vi "Fetch Measurement (Multiple Point).vi"(0 "VISA resource name":refnum<visa-resource-name>, 5 "Timeout (10000 ms)":u32=10000, 11 "error in (no error)":errorcluster) -> (3 "Go":bool, 4 "VISA resource name out":refnum<visa-resource-name>, 6 "Measurements":dbl[](array[numeric]) format="%#_7g", 10 "Questionable Data":bool, 13 "High":bool, 14 "Low":bool, 15 "error out":errorcluster)   [LabVIEW 2017, in "ADCMT 6240.lvlib"]
doc: "Fetch measurements from the measurement data memory on the instrument."
uses:
  ADCMT 6240.lvlib
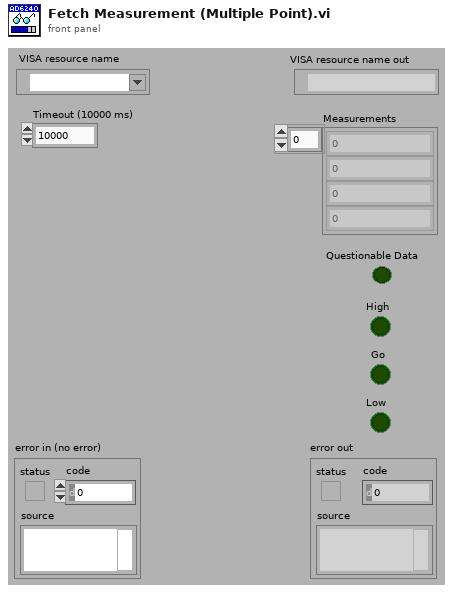
[diagram p1: front panel]
types:
  T1 = typedef "ADCMT 6240.lvlib/Extended User Data.ctl" = cluster{"Trigger Mode":u16, "Output Mode":u16, "Sample Count":i32, "Model":u16}
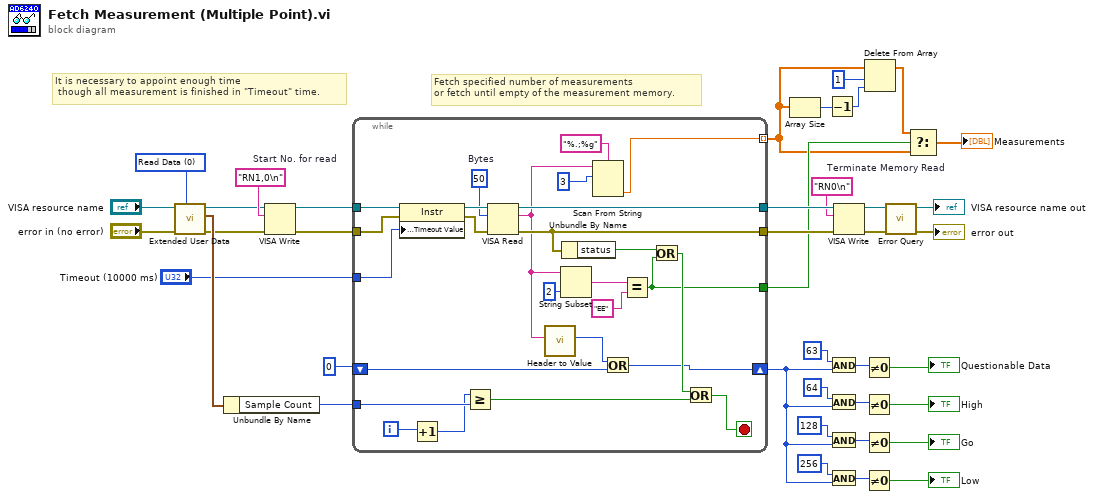
[diagram p0: block diagram]
diagram:
  w22 = "RN0\n"  # Terminate Memory Read
  w35 = u16 0 items=["Read Data", "Write Data", "Dispose of Data"] ("Action")
  w33 = "RN1,0\n"  # Start No. for read
  # "Fetch specified number of measurements\nor fetch until empty of the measurement memory."
  # "It is necessary to appoint enough time\n though all measurement is finished in \"Timeout\" time."
  n1 = call "Extended User Data.vi"("Action"=w35, "Error In (no error)"="error in (no error)", "VISA resource name in"="VISA resource name") -> ("Error Out"=w25:errorcluster, "User Data Out"=w34:T1, "VISA resource name out"=w26:refnum<visa-resource-name>)  [unwired: 6 in]
  n2 = Unbundle By Name ("名前でバンドル解除")(w34) -> ("Sample Count"=w24:i32)
  n3 = VISA Write ("VISA書き込み")(VISA resource name=w26, write buffer=w33, error in (no error)=w25) -> (VISA resource name out=w32:refnum<visa-resource-name>, error out=w31:errorcluster)  [unwired: 1 out]
  n4 = while "Whileループ" {
    tunnel: [w65] -> w30
    tunnel: [w60] -> w29
    tunnel: w32 -> [w62]
    tunnel: w31 -> [w61]
    tunnel: w24 -> [w56]
    shift-right: [w41] -> w5
    shift-left: 0 -> [w40]
    tunnel: "Timeout (10000 ms)" -> [w49]
    tunnel: [w46] -> w15 mode=indexing
    tunnel: [w45] -> w18
    i -> [w51]
    stop <- w55 stop-if-true
    w44 = u32 50  # Bytes
    n5 = property on="Property Node" class="Instr"(reference=w62, error in=w61, "General Settings:Timeout Value"=w49) -> (reference out=w64:refnum<visa-resource-name>, error out=w63:errorcluster)
    n6 = Increment ("インクリメント")(x=w51) -> (x+1=w50:i32)
    n7 = Greater Or Equal? ("以上?")(x=w50, y=w56) -> (x >= y?=w52:bool)
    n8 = VISA Read ("VISA読み取り")(VISA resource name=w64, byte count=w44, error in (no error)=w63) -> (VISA resource name out=w65:refnum<visa-resource-name>, read buffer=w43:string, error out=w60:errorcluster)  [unwired: 1 out]
    n9 = call "Header to Value.vi"("Header String (\"\")"=w43) -> ("Header Information"=w42:u32)  [unwired: 10 in]
    n10 = String Subset ("部分文字列")(string=w43, length (rest)=2) -> (substring=w58:string)  [unwired: 1 in]
    n11 = Unbundle By Name ("名前でバンドル解除")(w60) -> ("status"=w54:bool)
    n12 = Scan From String ("文字列からスキャン")(format string="%.;%g" ("Format String"), input string=w43, initial scan location=3) -> (output 1=w46:dbl)  [unwired: 2 in, 3 out]
    n13 = Or(x=w42, y=w40) -> (x .or. y?=w41:u32)
    n14 = Equal? ("等しい?")(x=w58, y="EE") -> (x = y?=w45:bool)
    n15 = Or(x=w54, y=w45) -> (x .or. y?=w53:bool)
    n16 = Or(x=w53, y=w52) -> (x .or. y?=w55:bool)
  }
  n17 = Array Size ("配列サイズ")(array=w15) -> (size(s)=w20:i32)
  n18 = Decrement ("デクリメント")(x=w20) -> (x-1=w19:i32)
  n19 = And(x=63, y=w5) -> (x .and. y?=w13:u32)
  n20 = And(x=64, y=w5) -> (x .and. y?=w11:u32)
  n21 = And(x=128, y=w5) -> (x .and. y?=w8:u32)
  n22 = And(x=256, y=w5) -> (x .and. y?=w7:u32)
  n23 = VISA Write ("VISA書き込み")(VISA resource name=w30, write buffer=w22, error in (no error)=w29) -> (VISA resource name out=w27:refnum<visa-resource-name>, error out=w28:errorcluster)  [unwired: 1 out]
  n24 = Not Equal To 0?(x=w13) -> (x != 0?=→"Questionable Data":bool)
  n25 = Not Equal To 0?(x=w11) -> (x != 0?=→"High":bool)
  n26 = Not Equal To 0?(x=w8) -> (x != 0?=→"Go":bool)
  n27 = Not Equal To 0?(x=w7) -> (x != 0?=→"Low":bool)
  n28 = Delete From Array ("配列から削除")(array=w15, length=1, index=w19) -> (array with subset deleted=w17:dbl[])  [unwired: 1 out]
  n29 = call "Error Query.vi"("error in (no error)"=w28, "VISA resource name"=w27) -> ("error out"=→"error out":errorcluster, "VISA resource name out"=→"VISA resource name out":refnum<visa-resource-name>)  [unwired: 6 in, 2 out]
  n30 = Select ("選択")(t=w17, s=w18, f=w15) -> (s? t:f=→"Measurements":dbl[])
